vi "RIMP.vi"(2 "Run uninterrupted?":bool, 3 "Device Category IN:":string(combo)="Mini" caption="Device Category:", 4 "Batch No. IN:":string caption="Batch No.:", 5 "Sensor Serial No. IN:":string caption="Sensor Serial No.:", 6 "DB Serial No. IN:":string caption="DB Serial No.:") -> (0 "Done!":bool)   [LabVIEW 2019]
doc: "Performs IV measurements according to ATLAS ITk Quality Control Specifications."
uses:
  InstrControl/SupplyControl/SupplyControl.lvclass
  general_VIs/globals/QC_RunInformation.vi
  InstrControl/ArduinoControl/ArduinoControl.lvclass
  general_VIs/globals/QC_MeasurementSetup.vi
  <vilib>/Analysis/NI_AALBase.lvlib
  InstrControl/InstrumentSetup.vi
  InstrControl/InstrControl.lvclass
  InstrControl/Switching/Switching.lvclass
panel:
  out "Measurement Configuration Tab":enum32{"IV Setup", "IV Scan"}(tab)
  in  "Set current limit?":bool
  in  "Current Limit [µA]":dbl=1000.0 min=0.0001 format="%.3f"
  in  "Measurement Configurations":bool
  in  "Initial volts [V] IN":dbl caption="Initial volts [V]"
  in  "Final volts [V] IN":dbl=-700.0 caption="Final volts [V]"
  in  "step [V] IN":dbl=10.0 caption="step [V]" format="%.1f"
  in  "step interval [s] IN":i32=10 caption="step interval [s]"
  in  "Continue":bool
  in  "Quit":bool
  out "RH":dbl[](array[numeric]) caption="RH [%]" format="%#.2f"
  out "Temp.":dbl[](array[numeric]) caption="Temp. [°C]" format="%#.2f"
  out "Current":dbl[](array[numeric]) caption="Current [nA]"
  out "Volts":dbl[](array[numeric]) caption="Volts [V]"
  out "step interval [s]":i32=10
  out "step [V]":dbl=10.0 format="%.1f"
  out "Final volts [V]":dbl=-700.0 format="%.1f"
  out "Initial volts [V]":dbl format="%.1f"
  out "Igraph":cluster{dbl[], dbl[]}(graph)
  in  "Scales":T1(ring)
  in  "Iscale":enum16{"nanoAmps", "microAmps", "milliAmps"}(ring)
  out "positive ramp?":bool
  out "DUT Description/Hardware Tab":enum32{"IV Setup", "IV Scan"}(tab)
  in  "Structure Name IN:":string caption="Structure Name:"
  in  "Switching":string(combo)="LXIPXI Switching"
  in  "Hardware Configurations":bool
  in  "User:":string(combo)="Xavi"
  in  "IV Supply":string(combo)="Keithley 2410"
  in  "Temperature":enum16{"Read Arduino", "Enter manually"}(ring)
  in  "Manufacturer:":string(combo)="Hamamatsu"
  out "Structure Name":string caption="Structure Name:"
  in  "abort":bool
  out "Device Category:":string
  out "DB Serial No.:":string
  out "Current Volts:":dbl format="%.2f"
  in  "quit (no save)":bool
  in  "Quit & Save":bool
  out "Bias On/Off:":bool
  out "STATUS 1":string
  out "Initiated:":string
  out "Sensor No.:":string
  out "No of steps":u32
  out "Current reading No.":u32
  out "Last reading at:":string
  # "University of\nCambridge"
  # "Strip Sensor QC: Implant Resistance"
  # "Vertical Scale:"
  # "Measurement Configuration"
  # "Scan parameters:"
  # "Last 5 readings:"
  # "n-4"
  # "n-3"
  # "n-2"
  # "n-1"
  # "n"
  # "DUT Description"
  # "Hardware"
  # "DUT & Test Description:"
  # "Current status:"
  # "Rdg No:"
  # "out of"
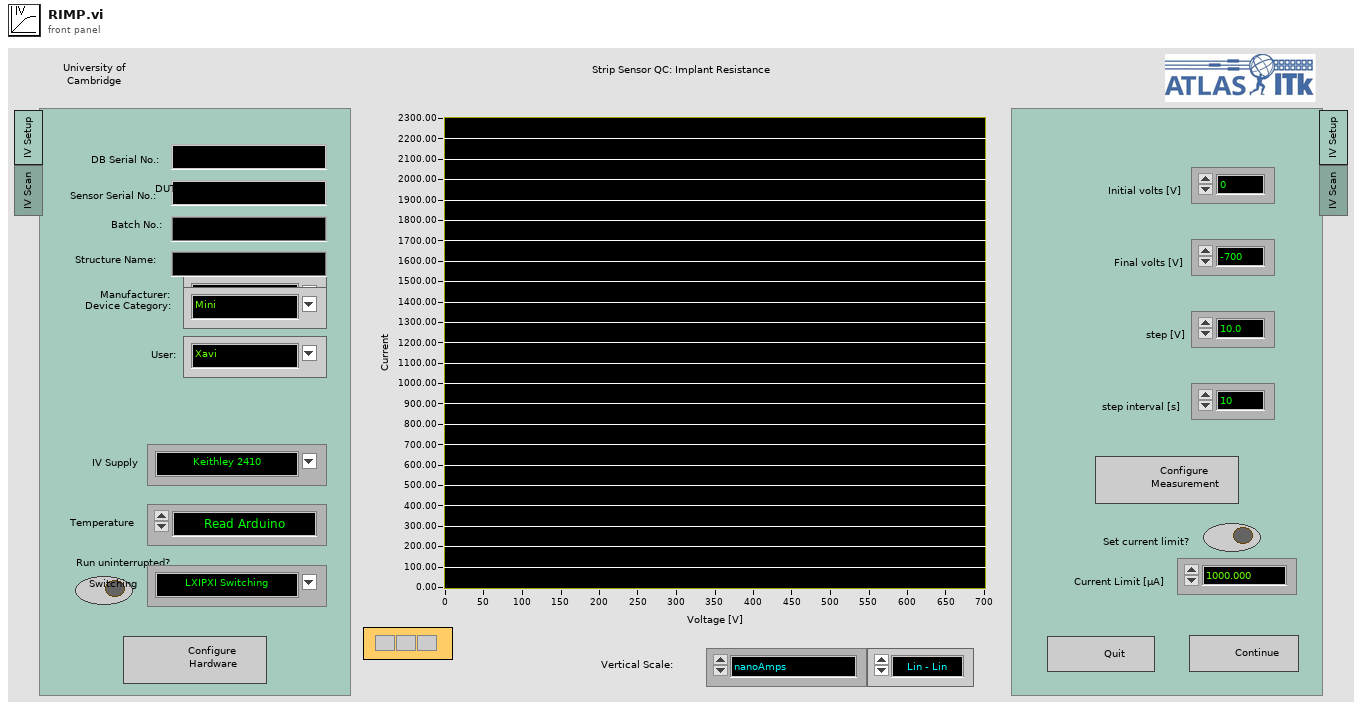
[diagram p1: front panel]
types:
  T1 = enum16{"Lin - Lin", "Log - Lin", "Lin - Log", "Log - log"}
  T2 = enum16{"Supply", "LCR", "Multimeter", "Switching"}
  T3 = enum16{"Reset", "Read Array", "Read Element", "Write Element", "Write Array", "Add Element", "Add Array"}
  T4 = enum16{"Reset", "Ground", "Striptest Bias", "Striptest SMU", "Striptest LCR", "IV", "CV", "Interstrip Cap", "Interstrip Res"}
  T5 = enum32{"IV", "CV", "Stability", "Striptest", "Cis", "Ris", "PTP"}
  T6 = cluster{"Supply":refnum<class "SupplyControl.lvclass">, "Initial Voltage [V]":dbl, "Final Voltage [V]":dbl, "Step Size [V]":dbl, "Step Interval [s]":i32, "Number Of Steps":u32, "Ramp down steps [V]":dbl, "Ramp down Interval [s]":i32, "Set Current Limit?":bool, "Current Limit [µA]":dbl, "Temperature Readout":enum16{"Read Arduino", "Enter manually"}, "Arduino":refnum<class "ArduinoControl.lvclass">, "Supply Name":string, "Switching":refnum<class "Switching.lvclass">, "Matrix used?":bool, "Matrix X Channels":cluster{"Bias Supply / SMU LO":i32, "Bias Supply / SMU HI":i32, "CV Box LO":i32, "CV Box HI":i32, "CV Box LO IN":i32, "CV Box HI IN":i32, "Volt meter LO":i32, "Volt meter HI":i32, "Mux1 C1":i32, "Mux1 C2":i32, "Mux2 C1":i32, "Mux2 C2":i32}, "Structure Name":string}
  T7 = cluster{"Sensor Serial No.:":string, "Wafer Serial No.:":string, "Batch:":string, "Manufacturer:":string, "Device Category:":string, "Database Serial No.:":string, "Date Initiated:":string, "Time Initiated:":string, "Test":string, "Instruments used:":string, "Probeplan used:":string, "End of Run comment:":string, "User:":string}
  T8 = cluster{"Institute":string, "Manufacturers":string[], "Devices":string[], "Serialnumbers Lookup DB":string, "Data directory":string, "Backup & screenshot directory":string, "List of known users":string[], "Measurement switch not used":bool, "Measurement Switch":string, "DUT Switch":string}
  T9 = cluster{"VISA address":refnum<visa-resource-name>, "T sensor":enum16{"SHT", "DS"}, "Arduino":refnum<class "ArduinoControl.lvclass">}
  T10 = cluster{"Supply":refnum<class "SupplyControl.lvclass">, "Initial Voltage [V]":dbl, "Final Voltage [V]":dbl, "Step Size [V]":dbl, "Step Interval [s]":i32, "Number Of Steps":u32, "Ramp down steps [V]":dbl, "Ramp down Interval [s]":i32, "hold steps":i32, "Set Current Limit?":bool, "Current Limit [µA]":dbl, "Temperature Readout":enum16{"Read Arduino", "Enter manually"}, "Arduino":refnum<class "ArduinoControl.lvclass">, "Supply Name":string, "V_breakdown Limit [V]":dbl, "Switching":refnum<class "Switching.lvclass">, "Matrix used?":bool, "Matrix X Channels":cluster{"Bias Supply / SMU LO":i32, "Bias Supply / SMU HI":i32, "CV Box LO":i32, "CV Box HI":i32, "CV Box LO IN":i32, "CV Box HI IN":i32, "Volt meter LO":i32, "Volt meter HI":i32, "Mux1 C1":i32, "Mux1 C2":i32, "Mux2 C1":i32, "Mux2 C2":i32}}
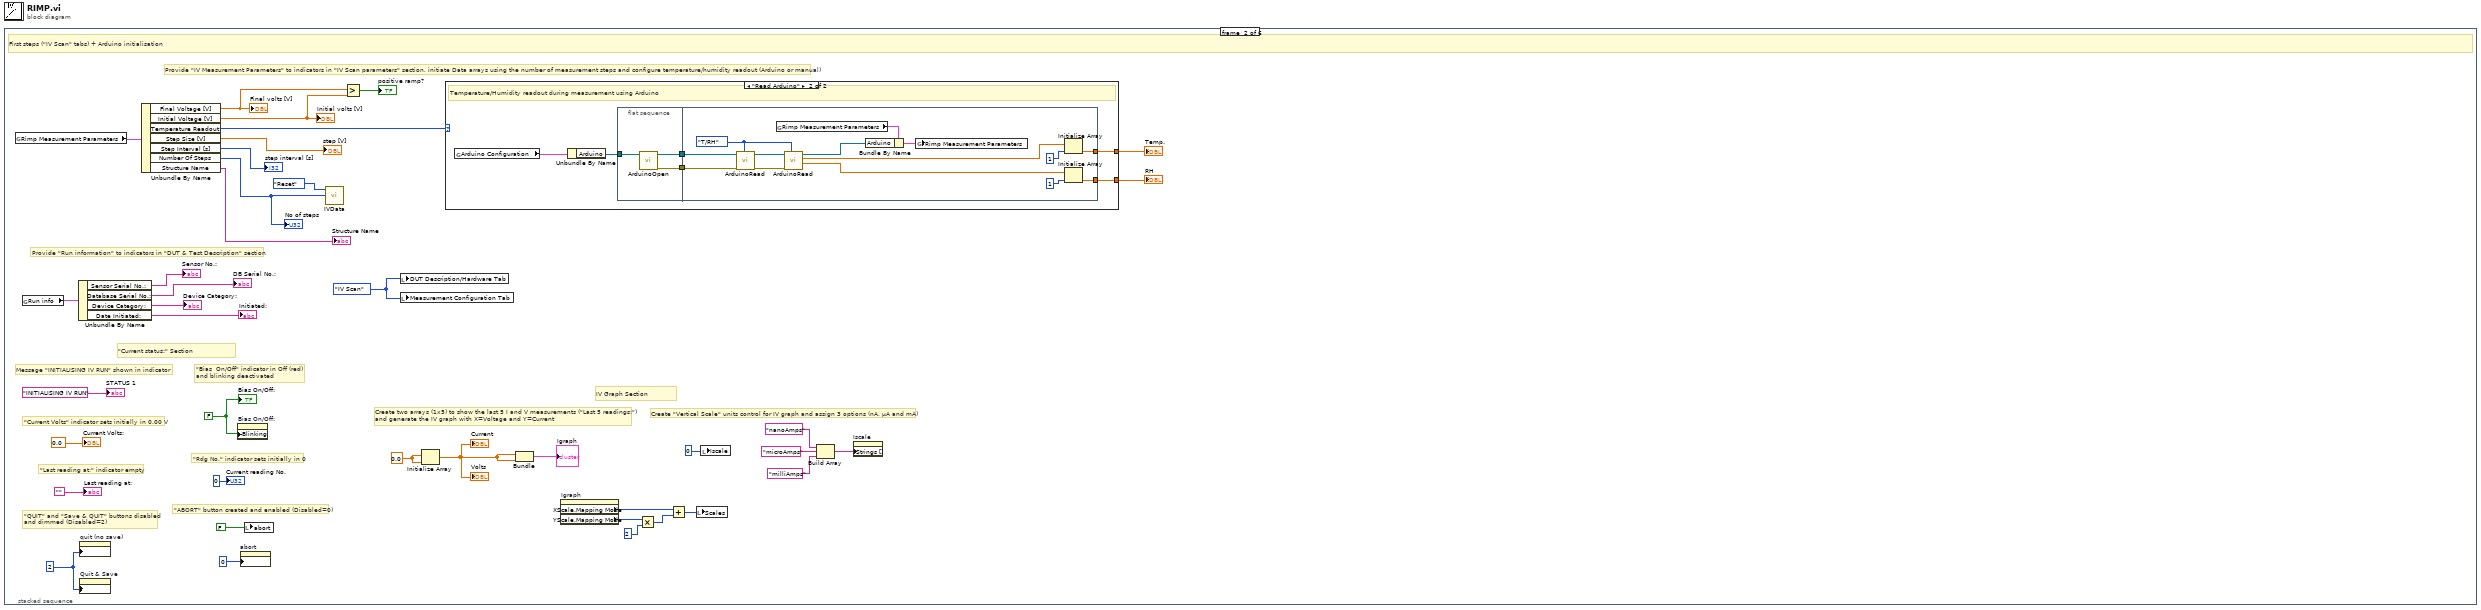
[diagram p0: block diagram]
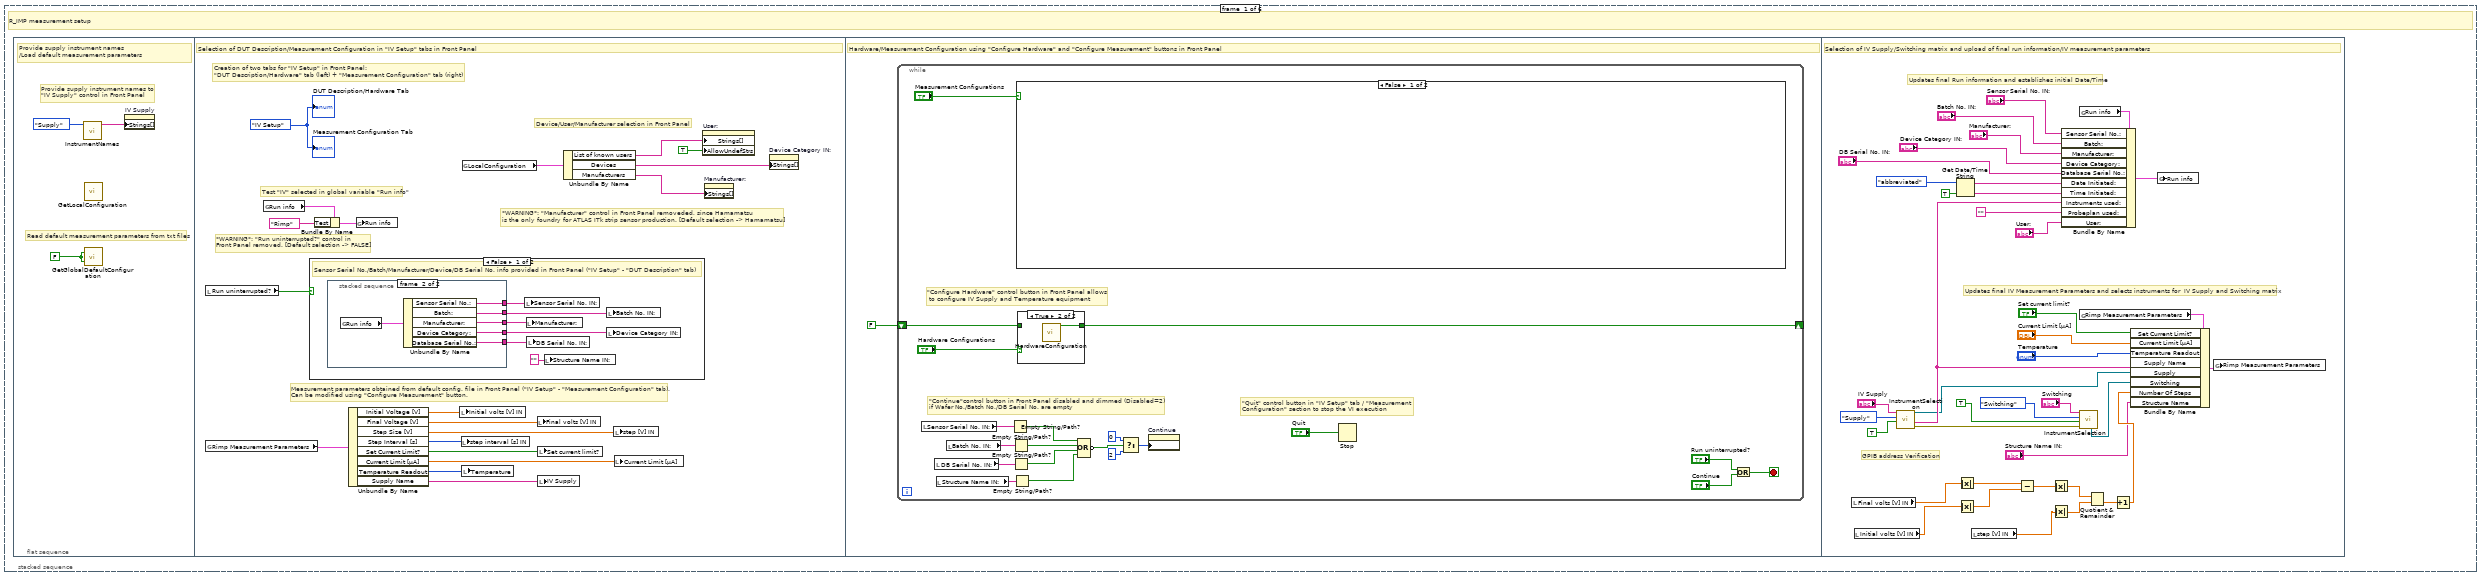
[diagram p2: hidden frame]
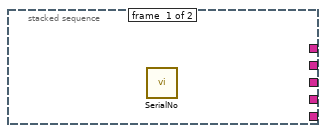
[diagram p3: hidden frame]
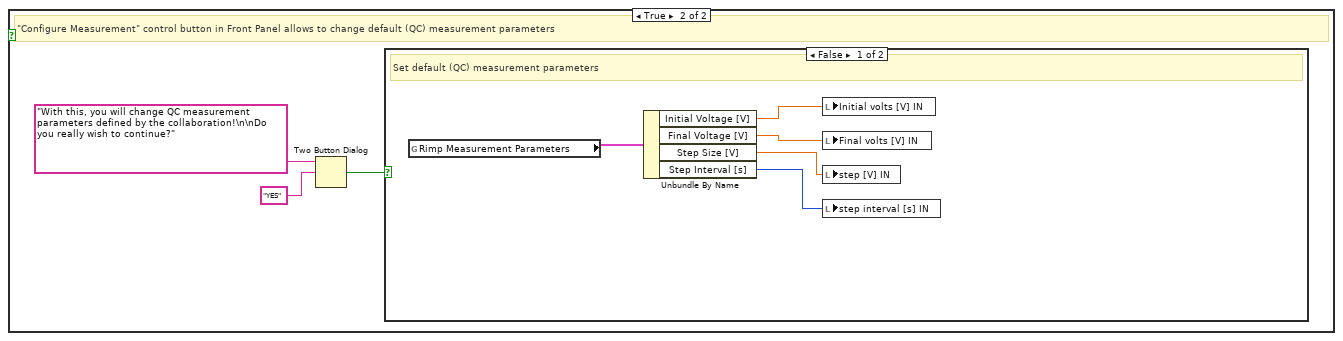
[diagram p5: hidden frame]
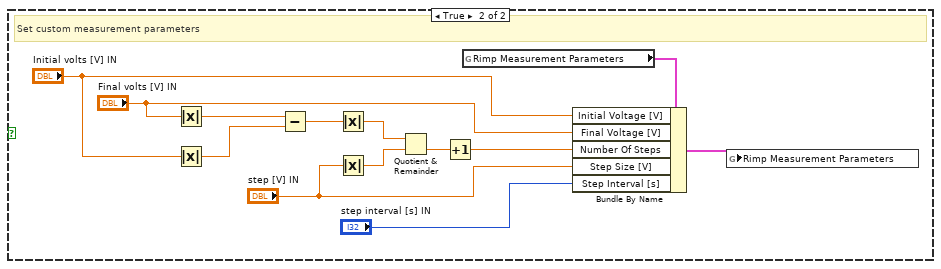
[diagram p6: hidden frame]
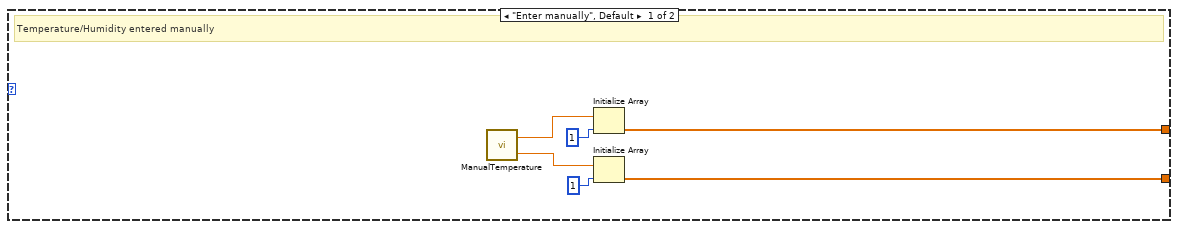
[diagram p8: hidden frame]
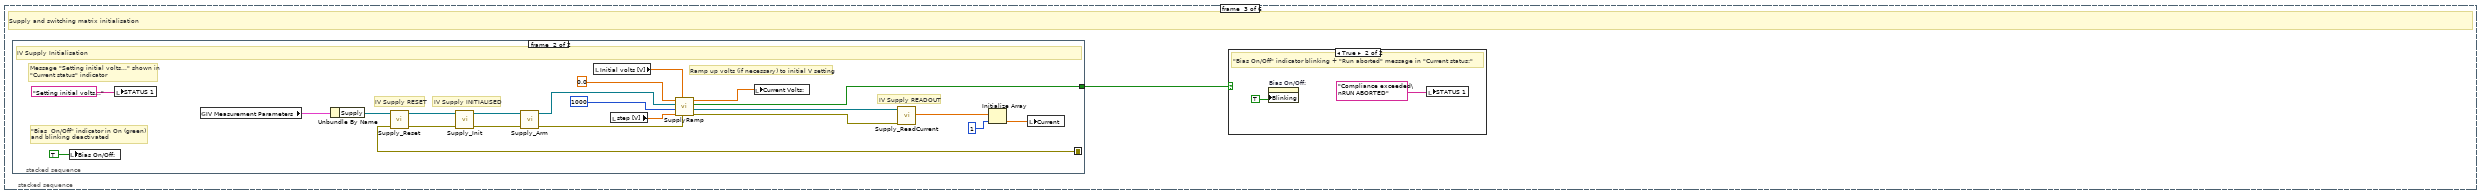
[diagram p9: hidden frame]
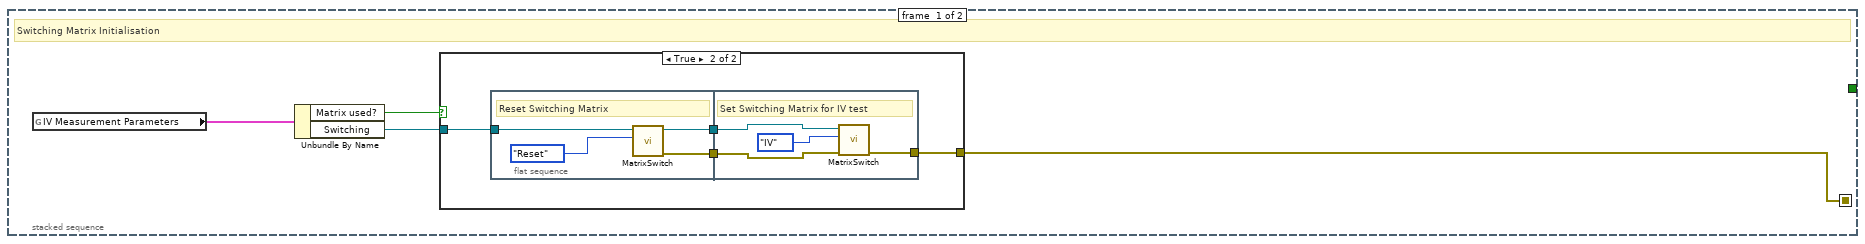
[diagram p10: hidden frame]
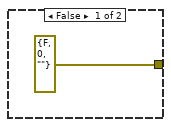
[diagram p11: hidden frame]
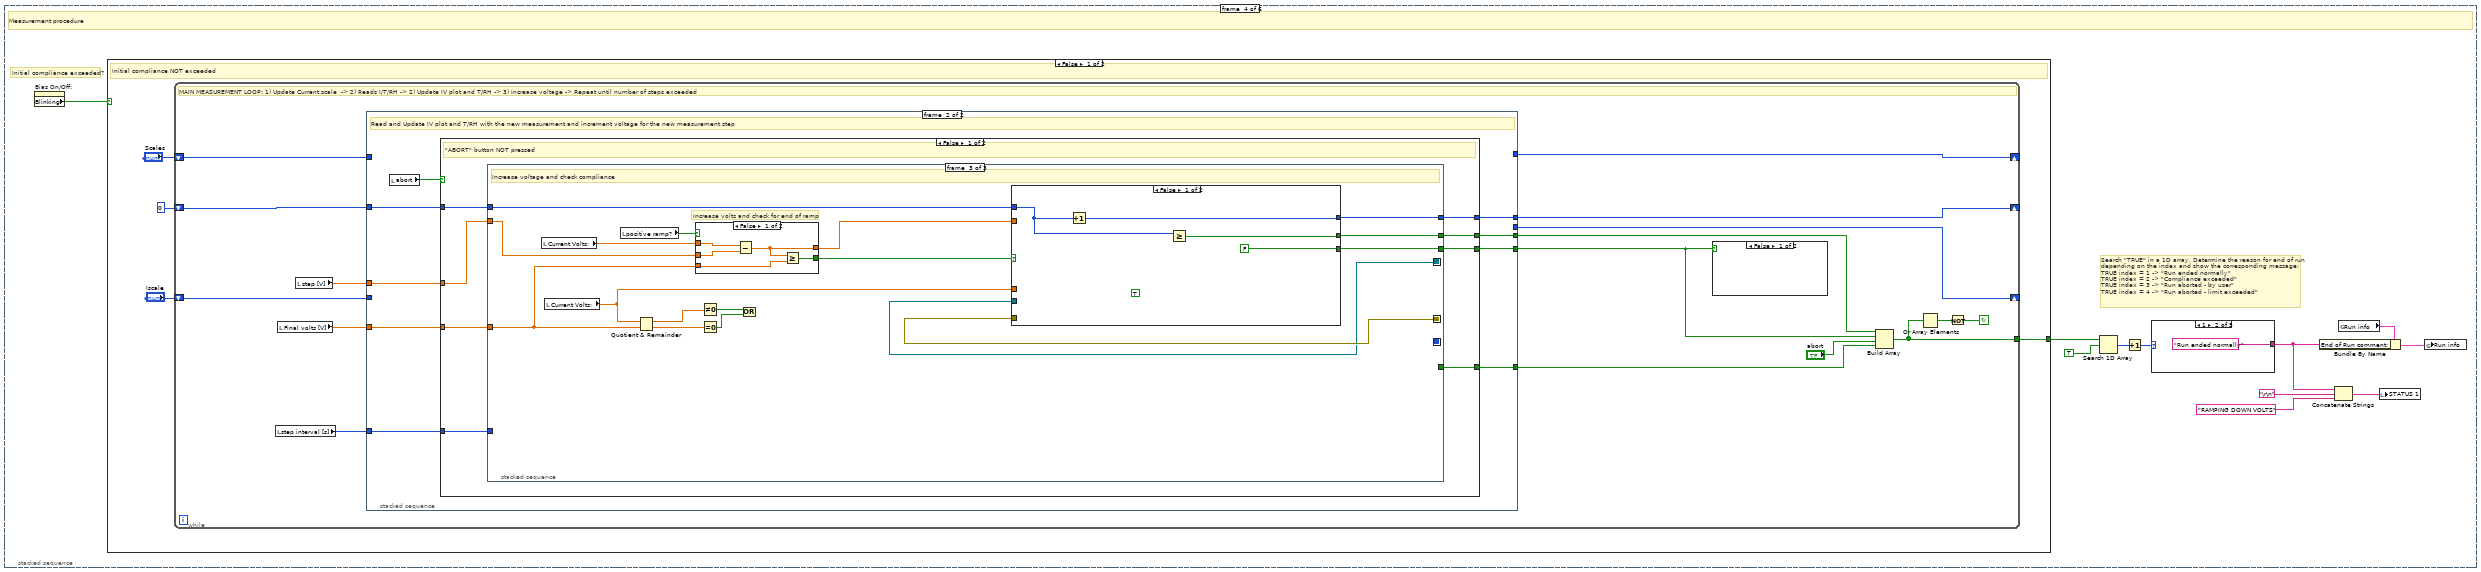
[diagram p13: hidden frame]
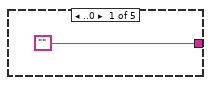
[diagram p14: hidden frame]
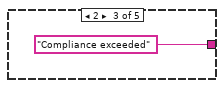
[diagram p15: hidden frame]
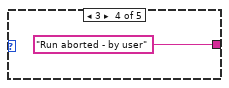
[diagram p16: hidden frame]
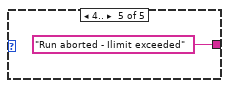
[diagram p17: hidden frame]
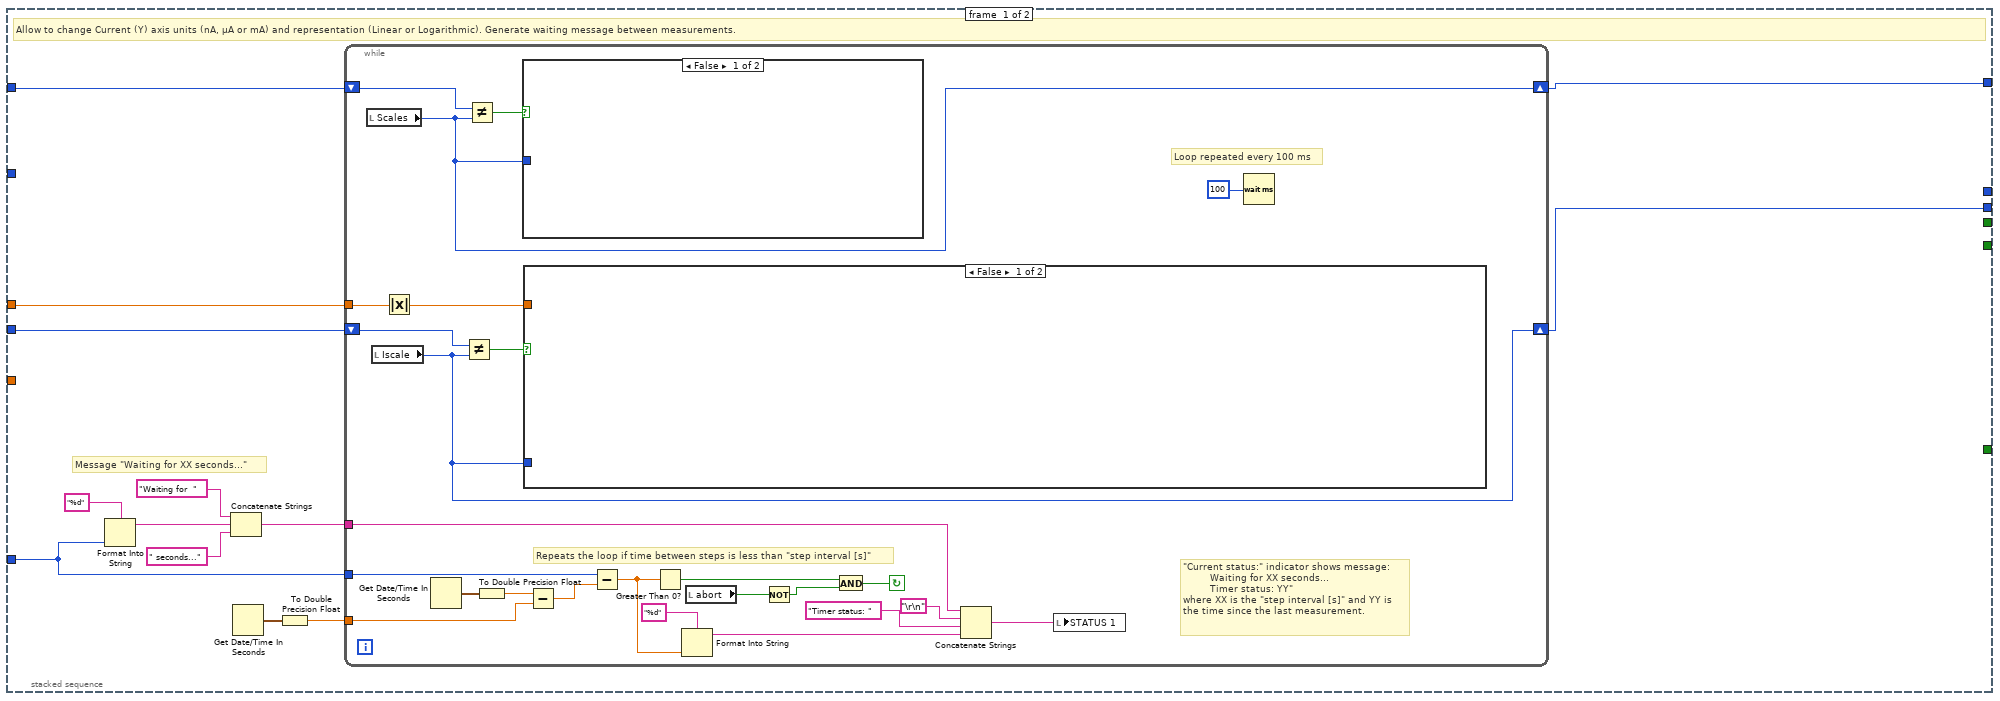
[diagram p18: hidden frame]
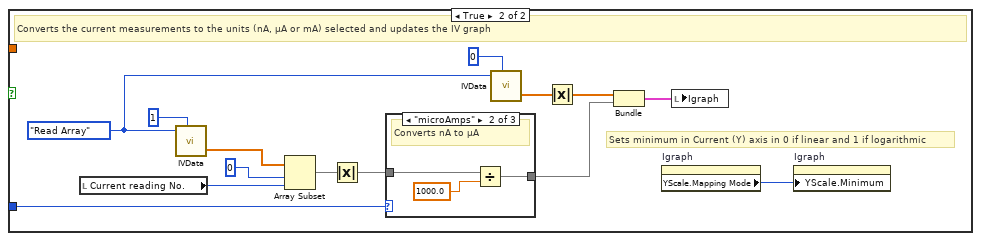
[diagram p19: hidden frame]
diagram:
  n1 = stacked-sequence {
    frame #0 {
      # "R_IMP measurement setup"
      n2 = flat-sequence {
        frame #0 {
          w3 = FALSE
          # "Read default measurement parameters from txt files"
          # "Provide supply instrument names to \n\"IV Supply\" control in Front Panel"
          # "Provide supply instrument names\n/Load default measurement parameters"
          n3 = call "InstrumentNames.vi"("Instrument type"=T2."Supply") -> ("Instrument names"=w1:string[])  [unwired: 9 in, 1 out]
          n4 = call "GetLocalConfiguration.vi"() -> ()  [unwired: 3 in, 1 out]
          n5 = call "GetGlobalDefaultConfiguration.vi"("DO NOT override instruments"=w3, "Read defaults?"=w3) -> ()  [unwired: 1 in, 1 out]
          n6 = property on="IV Supply" class="CmbBox"("Strings[]"=w1) -> ()  [unwired: 2 in, 2 out]
        }
        frame #1 {
          w11 = enum32{"IV Setup", "IV Scan"}."IV Setup" ("Tab Control")
          # "Device/User/Manufacturer selection in Front Panel"
          # "*WARNING*: \"Manufacturer\" control in Front Panel removeded, since Hamamatsu \nis the only foundry for ATLAS ITk strip sensor production. [Default selection -> Hamamatsu]"
          # "Measurement parameters obtained from default config. file in Front Panel (\"IV Setup\" - \"Measurement Configuration\" tab).\nCan be modified using \"Configure Measurement\" button."
          # "Test \"IV\" selected in global variable \"Run info\""
          # "Creation of two tabs for \"IV Setup\" in Front Panel:\n\"DUT Description/Hardware\" tab (left) + \"Measurement Configuration\" tab (right)"
          # "*WARNING*: \"Run uninterrupted?\" control in \nFront Panel removed. [Default selection -> FALSE]"
          # "Selection of DUT Description/Measurement Configuration in \"IV Setup\" tabs in Front Panel"
          n7 = local read "Run uninterrupted?"() -> (w14:bool)
          n8 = global read "QC_MeasurementSetup.vi" "Rimp Measurement Parameters"() -> (w20:T6)
          n9 = global read "QC_RunInformation.vi" "Run info"() -> (w13:T7)
          n10 = case shown="False" w14 {
            frame False {
              # "Sensor Serial No./Batch/Manufacturer/Device/DB Serial No. info provided in Front Panel (\"IV Setup\" - \"DUT Description\" tab)"
              n11 = stacked-sequence {
                tunnel: [_ w34] -> w27
                tunnel: [_ w33] -> w26
                tunnel: [_ w32] -> w25
                tunnel: [_ w31] -> w28
                tunnel: [_ w29] -> w24
                frame #0 {
                  n12 = call "SerialNo.vi"() -> ()  [unwired: 5 in, 1 out]
                }
                frame #1 {
                  n13 = global read "QC_RunInformation.vi" "Run info"() -> (w30:T7)
                  n14 = Unbundle By Name(w30) -> ("Sensor Serial No.:"=w34:string, "Batch:"=w33:string, "Manufacturer:"=w32:string, "Device Category:"=w31:string, "Database Serial No.:"=w29:string)
                }
              }
              n15 = local write "Sensor Serial No. IN:"(w27) -> ()
              n16 = local write "Manufacturer:"(w25) -> ()
              n17 = local write "DB Serial No. IN:"(w24) -> ()
              n18 = local write "Structure Name IN:"("" ("Structure Name IN:")) -> ()
              n19 = local write "Batch No. IN:"(w26) -> ()
              n20 = local write "Device Category IN:"(w28) -> ()
            }
            frame True {
            }
          }
          n21 = Bundle By Name(cluster=w13, "Test"="Rimp") -> (w12:T7)
          n22 = Unbundle By Name(w20) -> ("Initial Voltage [V]"=w9:dbl, "Final Voltage [V]"=w8:dbl, "Step Size [V]"=w7:dbl, "Step Interval [s]"=w10:i32, "Set Current Limit?"=w19:bool, "Current Limit [µA]"=w18:dbl, "Temperature Readout"=w22:enum16{"Read Arduino", "Enter manually"}, "Supply Name"=w21:string)
          n23 = global write "QC_RunInformation.vi" "Run info"(w12) -> ()
          n24 = local write "Initial volts [V] IN"(w9) -> ()
          n25 = local write "step interval [s] IN"(w10) -> ()
          n26 = local write "Temperature"(w22) -> ()
          n27 = global read "QC_RunInformation.vi" "LocalConfiguration"() -> (w17:T8)
          n28 = local write "Final volts [V] IN"(w8) -> ()
          n29 = local write "Set current limit?"(w19) -> ()
          n30 = local write "IV Supply"(w21) -> ()
          n31 = Unbundle By Name(w17) -> ("List of known users"=w16:string[], "Devices"=w6:string[], "Manufacturers"=w5:string[])
          n32 = local write "step [V] IN"(w7) -> ()
          n33 = local write "Current Limit [µA]"(w18) -> ()
          n34 = property on="User:" class="CmbBox"("Strings[]"=w16, "AllowUndefStrs"=TRUE) -> ()  [unwired: 2 in, 2 out]
          n35 = property on="Manufacturer:" class="CmbBox"("Strings[]"=w5) -> ()  [unwired: 2 in, 2 out]
          n36 = property on="Device Category IN:" class="CmbBox"("Strings[]"=w6) -> ()  [unwired: 2 in, 2 out]
          "DUT Description/Hardware Tab" <- w11
          "Measurement Configuration Tab" <- w11
        }
        frame #2 {
          # "Hardware/Measurement Configuration using \"Configure Hardware\" and \"Configure Measurement\" buttons in Front Panel"
          n37 = while {
            shift-right: [w45] -> _
            shift-left: FALSE -> [w44]
            stop <- w41 stop-if-true
            # "\"Continue\"control button in Front Panel disabled and dimmed (Disabled=2) \nif Wafer No./Batch No./DB Serial No. are empty"
            # "\"Configure Hardware\" control button in Front Panel allows\n to configure IV Supply and Temperature equipment"
            # "\"Quit\" control button in \"IV Setup\" tab / \"Measurement \nConfiguration\" section to stop the VI execution"
            n38 = local read "Sensor Serial No. IN:"() -> (w54:string)
            n39 = local read "DB Serial No. IN:"() -> (w39:string)
            n40 = local read "Structure Name IN:"() -> (w37:string)
            n41 = local read "Batch No. IN:"() -> (w47:string)
            n42 = Empty String/Path?(string/path=w54) -> (empty?=w53:bool)
            n43 = Empty String/Path?(string/path=w47) -> (empty?=w46:bool)
            n44 = Empty String/Path?(string/path=w39) -> (empty?=w38:bool)
            n45 = Empty String/Path?(string/path=w37) -> (empty?=w36:bool)
            n46 = case shown="False" "Measurement Configurations" {
              frame False {
              }
              frame True {
                # "\"Configure Measurement\" control button in Front Panel allows to change default (QC) measurement parameters"
                n47 = Two Button Dialog(message="With this, you will change QC measurement parameters defined by the collaboration!\n\nDo you really wish to continue?", 2:"YES") -> (T button?=w56:bool)  [unwired: 1 in]
                n48 = case shown="False" w56 {
                  frame False {
                    # "Set default (QC) measurement parameters"
                    n49 = global read "QC_MeasurementSetup.vi" "Rimp Measurement Parameters"() -> (w63:T6)
                    n50 = Unbundle By Name(w63) -> ("Initial Voltage [V]"=w61:dbl, "Final Voltage [V]"=w62:dbl, "Step Size [V]"=w60:dbl, "Step Interval [s]"=w59:i32)
                    n51 = local write "Initial volts [V] IN"(w61) -> ()
                    n52 = local write "Final volts [V] IN"(w62) -> ()
                    n53 = local write "step [V] IN"(w60) -> ()
                    n54 = local write "step interval [s] IN"(w59) -> ()
                  }
                  frame True {
                    # "Set custom measurement parameters"
                    n55 = Absolute Value(x="Final volts [V] IN") -> (abs(x)=w74:dbl)
                    n56 = Absolute Value(x="Initial volts [V] IN") -> (abs(x)=w73:dbl)
                    n57 = Subtract(x=w74, y=w73) -> (x-y=w68:dbl)
                    n58 = Absolute Value(x=w68) -> (abs(x)=w70:dbl)
                    n59 = Absolute Value(x="step [V] IN") -> (abs(x)=w69:dbl)
                    n60 = Quotient & Remainder(x=w70, y=w69) -> (floor(x/y)=w67:dbl)  [unwired: 1 out]
                    n61 = Increment(x=w67) -> (x+1=w66:dbl)
                    n62 = global read "QC_MeasurementSetup.vi" "Rimp Measurement Parameters"() -> (w76:T6)
                    n63 = Bundle By Name(cluster=w76, "Initial Voltage [V]"="Initial volts [V] IN", "Final Voltage [V]"="Final volts [V] IN", "Number Of Steps"=w66, "Step Size [V]"="step [V] IN", "Step Interval [s]"="step interval [s] IN") -> (w75:T6)
                    n64 = global write "QC_MeasurementSetup.vi" "Rimp Measurement Parameters"(w75) -> ()
                  }
                }
              }
            }
            n65 = case shown="True" "Hardware Configurations" {
              tunnel: [w77 w78] -> w45
              tunnel: w44 -> [w77 _]
              frame False {
              }
              frame True {
                n66 = call "HardwareConfiguration.vi"() -> ("configured?"=w78:bool)  [unwired: 11 in]
              }
            }
            n67 = Compound Arithmetic op=OR(w53, w46, w38, w36) -> (invert w52:bool)
            n68 = Select(t=0, s=w52, f=2) -> (s? t:f=w49:i32)
            n69 = property on="Continue" class="Bool"("DisabledEnum"=w49) -> ()  [unwired: 2 in, 2 out]
            n70 = Stop(stop? (T)="Quit") -> ()
            n71 = Or(x="Run uninterrupted?", y="Continue") -> (x .or. y?=w41:bool)
          }
        }
        frame #3 {
          # "GPIB address Verification"
          # "Updates final IV Measurement Parameters and selects instruments for  IV Supply and Switching matrix"
          # "Updates final Run information and establishes initial Date/Time"
          # "Selection of IV Supply/Switching matrix and upload of final run information/IV measurement parameters"
          n72 = local read "Final volts [V] IN"() -> (w81:dbl)
          n73 = local read "Initial volts [V] IN"() -> (w82:dbl)
          n74 = call "InstrumentSelection.vi"("Verify GPIB address"=TRUE, "Instrument type"=T2."Supply", "Instrument name IN"="IV Supply") -> ("error out"=w100:errorcluster, "Instrument name OUT"=w103:string, "Supply"=w102:refnum<class "SupplyControl.lvclass">)  [unwired: 3 in, 3 out]
          n75 = Get Date/Time String(date format (0)=enum16{"short", "long", "abbreviated"}."abbreviated", want seconds? (F)=TRUE) -> (date string=w93:string, time string=w92:string)  [unwired: 1 in]
          n76 = Absolute Value(x=w81) -> (abs(x)=w89:dbl)
          n77 = Absolute Value(x=w82) -> (abs(x)=w88:dbl)
          n78 = local read "step [V] IN"() -> (w83:dbl)
          n79 = Subtract(x=w89, y=w88) -> (x-y=w85:dbl)
          n80 = Absolute Value(x=w85) -> (abs(x)=w87:dbl)
          n81 = Absolute Value(x=w83) -> (abs(x)=w86:dbl)
          n82 = global read "QC_RunInformation.vi" "Run info"() -> (w111:T7)
          n83 = Bundle By Name(cluster=w111, "Sensor Serial No.:"="Sensor Serial No. IN:", "Batch:"="Batch No. IN:", "Manufacturer:"="Manufacturer:", "Device Category:"="Device Category IN:", "Database Serial No.:"="DB Serial No. IN:", "Date Initiated:"=w93, "Time Initiated:"=w92, "Instruments used:"=w103, "Probeplan used:"="", "User:"="User:") -> (w110:T7)
          n84 = global read "QC_MeasurementSetup.vi" "Rimp Measurement Parameters"() -> (w116:T6)
          n85 = call "InstrumentSelection.vi"("error in (no error)"=w100, "Verify GPIB address"=TRUE, "Instrument type"=T2."Switching", "Instrument name IN"="Switching") -> ("Switching"=w99:refnum<class "Switching.lvclass">)  [unwired: 2 in, 5 out]
          n86 = Quotient & Remainder(x=w87, y=w86) -> (floor(x/y)=w84:dbl)  [unwired: 1 out]
          n87 = Increment(x=w84) -> (x+1=w80:dbl)
          n88 = Bundle By Name(cluster=w116, "Set Current Limit?"="Set current limit?", "Current Limit [µA]"="Current Limit [µA]", "Temperature Readout"="Temperature", "Supply Name"=w103, "Supply"=w102, "Switching"=w99, "Number Of Steps"=w80, "Structure Name"="Structure Name IN:") -> (w117:T6)
          n89 = global write "QC_RunInformation.vi" "Run info"(w110) -> ()
          n90 = global write "QC_MeasurementSetup.vi" "Rimp Measurement Parameters"(w117) -> ()
        }
      }
    }
    frame #1 {
      w125 = enum32{"IV Setup", "IV Scan"}."IV Scan" ("Tab Control")
      w140 = 2
      w146 = 0.0
      w139 = FALSE ("Visible")
      # "IV Graph Section"
      # "\"Current status:\" Section"
      # "Create two arrays (1x5) to show the last 5 I and V measurements (\"Last 5 readings:\") \nand generate the IV graph with X=Voltage and Y=Current"
      # "\"Bias  On/Off\" indicator in Off (red)\nand blinking deactivated"
      # "\"Rdg No.\" indicator sets initially in 0"
      # "\"ABORT\" button created and enabled (Disabled=0)"
      # "\"Current Volts\" indicator sets initially in 0.00 V"
      # "\"Last reading at:\" indicator empty"
      # "\"QUIT\" and \"Save & QUIT\" buttons disabled\nand dimmed (Disabled=2)"
      # "Message \"INITIALISING IV RUN\" shown in indicator"
      # "Create \"Vertical Scale\" units control for IV graph and assign 3 options (nA, µA and mA)"
      # "Provide \"Run information\" to indicators in \"DUT & Test Description\" section"
      # "Provide \"IV Measurement Parameters\" to indicators in \"IV Scan parameters\" section, initiate Data arrays using the number of measurement steps and configure temperature/humidity readout (Arduino or manual)"
      # "First steps (\"IV Scan\" tabs) + Arduino initialisation"
      n91 = global read "QC_MeasurementSetup.vi" "Rimp Measurement Parameters"() -> (w130:T6)
      n92 = global read "QC_RunInformation.vi" "Run info"() -> (w155:T7)
      n93 = Unbundle By Name(w155) -> ("Sensor Serial No.:"=→"Sensor No.:":string, "Database Serial No.:"=→"DB Serial No.:":string, "Device Category:"=→"Device Category:":string, "Date Initiated:"=→"Initiated:":string)
      n94 = property on="quit (no save)" class="Bool"("DisabledEnum"=w140) -> ()  [unwired: 2 in, 2 out]
      n95 = property on="Quit & Save" class="Bool"("DisabledEnum"=w140) -> ()  [unwired: 2 in, 2 out]
      n96 = Unbundle By Name(w130) -> ("Final Voltage [V]"=w121:dbl, "Initial Voltage [V]"=w122:dbl, "Temperature Readout"=w123:enum16{"Read Arduino", "Enter manually"}, "Step Size [V]"=→"step [V]":dbl, "Step Interval [s]"=→"step interval [s]":i32, "Number Of Steps"=w119:u32, "Structure Name"=→"Structure Name":string)
      "No of steps" <- w119
      "Initial volts [V]" <- w122
      "Final volts [V]" <- w121
      n97 = property on="Bias On/Off:" class="Bool (strict)"("Blinking"=w139) -> ()  [unwired: 2 in, 2 out]
      n98 = property on="abort" class="Bool (strict)"("DisabledEnum"=0) -> ()  [unwired: 2 in, 2 out]
      n99 = local write "abort"(FALSE) -> ()
      n100 = call "IVData.vi"("Action"=T3."Reset", "Array Size / Index"=w119) -> ()  [unwired: 3 in, 2 out]
      n101 = Greater?(x=w121, y=w122) -> (0:→"positive ramp?":bool)
      n102 = local write "DUT Description/Hardware Tab"(w125) -> ()
      n103 = local write "Measurement Configuration Tab"(w125) -> ()
      n104 = Initialize Array(w146, w146) -> (w126:dbl[])
      "Volts" <- w126
      "Current" <- w126
      n105 = case shown="\"Read Arduino\"" w123 {
        tunnel: [w161 w168] -> w143
        tunnel: [w158 w167] -> w131
        frame "Enter manually", Default {
          # "Temperature/Humidity entered manually"
          n106 = call "ManualTemperature.vi"() -> ("Humidity [%] out"=w157:dbl, "Temperature [°C] out"=w162:dbl)
          n107 = Initialize Array(w162, 1) -> (w161:dbl[])
          n108 = Initialize Array(w157, 1) -> (w158:dbl[])
        }
        frame "Read Arduino" {
          # "Temperature/Humidity readout during measurement using Arduino"
          n109 = global read "InstrumentSetup.vi" "Arduino Configuration"() -> (w164:T9)
          n110 = Unbundle By Name(w164) -> ("Arduino"=w163:refnum<class "ArduinoControl.lvclass">)
          n111 = flat-sequence {
            tunnel: [w169] -> w166
            tunnel: [w171] -> w165
            tunnel: w163 -> [w170]
            tunnel: [w185] -> w168
            tunnel: [w182] -> w167
            tunnel: w166 -> [w176]
            tunnel: w165 -> [w175]
            frame #0 {
              n112 = call "ArduinoOpen.vi"("ArduinoControl in"=w170) -> ("error out"=w171:errorcluster, "ArduinoControl out"=w169:refnum<class "ArduinoControl.lvclass">)  [unwired: 9 in]
            }
            frame #1 {
              w172 = enum16{"T/RH", "Interlock", "Edgesense"}."T/RH" ("Arduino function")
              n113 = call "ArduinoRead.vi"("Arduino function"=w172, "error in (no error)"=w175, "ArduinoControl in"=w176) -> ("error out"=w174:errorcluster, "ArduinoControl out"=w173:refnum<class "ArduinoControl.lvclass">)  [unwired: 3 in, 4 out]
              n114 = global read "QC_MeasurementSetup.vi" "Rimp Measurement Parameters"() -> (w178:T6)
              n115 = call "ArduinoRead.vi"("Arduino function"=w172, "error in (no error)"=w174, "ArduinoControl in"=w173) -> ("rel. Humidity [%]"=w180:dbl, "Temperature [°C]"=w181:dbl, "ArduinoControl out"=w179:refnum<class "ArduinoControl.lvclass">)  [unwired: 3 in, 3 out]
              n116 = Bundle By Name(cluster=w178, "Arduino"=w179) -> (w177:T6)
              n117 = global write "QC_MeasurementSetup.vi" "Rimp Measurement Parameters"(w177) -> ()
              n118 = Initialize Array(w181, 1) -> (w185:dbl[])
              n119 = Initialize Array(w180, 1) -> (w182:dbl[])
            }
          }
        }
      }
      "Temp." <- w143
      "RH" <- w131
      n120 = Bundle(w126, w126) -> (→"Igraph":cluster{dbl[], dbl[]})  [unwired: 1 in]
      n121 = property on="Igraph" class="XYGraph (strict)"() -> ("XScale.Mapping Mode"=w134:u8, "YScale.Mapping Mode"=w133:u8)  [unwired: 2 in, 2 out]
      n122 = Multiply(x=w133, y=2) -> (x*y=w136:i32)
      n123 = Add(x=w134, y=w136) -> (x+y=w132:i32)
      n124 = local write "Scales"(w132) -> ()
      n125 = local write "Iscale"(u16 0 ("Scale")) -> ()
      n126 = Build Array("nanoAmps", "microAmps", "milliAmps") -> (w152:string[])
      n127 = property on="Iscale" class="Enum (strict)"("Strings []"=w152) -> ()  [unwired: 2 in, 2 out]
      "STATUS 1" <- "INITIALISING IV RUN"
      "Bias On/Off:" <- w139
      "Last reading at:" <- ""
      "Current reading No." <- u32 0 ("Current reading No.")
      "Current Volts:" <- 0.0 ("Current Volts:")
    }
    frame #2 {
      # "Supply and switching matrix initialisation"
      n128 = stacked-sequence {
        seq-local: [w188 _] -> [_ w204]
        tunnel: [_ w205] -> w186
        frame #0 {
          # "Switching Matrix Initialisation"
          n129 = global read "QC_MeasurementSetup.vi" "IV Measurement Parameters"() -> (w187:T10)
          n130 = Unbundle By Name(w187) -> ("Matrix used?"=w190:bool, "Switching"=w189:refnum<class "Switching.lvclass">)
          n131 = case shown="True" w190 {
            tunnel: w189 -> [_ w192]
            tunnel: [errorcluster {"status"=FALSE, "code"=0, "source"=""} ("error constant") w193] -> w188
            frame False {
            }
            frame True {
              n132 = flat-sequence {
                tunnel: [w199] -> w195
                tunnel: [w198] -> w194
                tunnel: w192 -> [w197]
                tunnel: w195 -> [w203]
                tunnel: w194 -> [w202]
                tunnel: [w201] -> w193
                frame #0 {
                  # "Reset Switching Matrix"
                  n133 = call-dynamic "MatrixSwitch.vi"("Action"=T4."Reset", "Switching in"=w197) -> ("error out"=w199:errorcluster, "Switching out"=w198:refnum<class "Switching.lvclass">)  [unwired: 7 in, 1 out]
                }
                frame #1 {
                  # "Set Switching Matrix for IV test"
                  n134 = call-dynamic "MatrixSwitch.vi"("error in (no error)"=w203, "Action"=T4."IV", "Switching in"=w202) -> ("error out"=w201:errorcluster)  [unwired: 6 in, 2 out]
                }
              }
            }
          }
        }
        frame #1 {
          # "IV Supply READOUT"
          # "IV Supply INITIALISED"
          # "IV Supply RESET"
          # "Message \"Setting initial volts...\" shown in \n\"Current status\" indicator"
          # "\"Bias  On/Off\" indicator in On (green)\nand blinking deactivated"
          # "Ramp up volts (if necessary) to initial V setting"
          # "IV Supply Initialisation"
          n135 = local write "Bias On/Off:"(TRUE ("Compliance?")) -> ()
          n136 = local write "STATUS 1"("Setting initial volts..." ("STATUS 1")) -> ()
          n137 = global read "QC_MeasurementSetup.vi" "IV Measurement Parameters"() -> (w221:T10)
          n138 = Unbundle By Name(w221) -> ("Supply"=w218:refnum<class "SupplyControl.lvclass">)
          n139 = call-dynamic "Supply_Reset.vi"("error in (no error)"=w204, "SupplyControl in"=w218) -> ("error out"=w223:errorcluster, "SupplyControl out"=w225:refnum<class "SupplyControl.lvclass">)  [unwired: 8 in]
          n140 = call-dynamic "Supply_Init.vi"("error in (no error)"=w223, "SupplyControl in"=w225) -> ("error out"=w222:errorcluster, "SupplyControl out"=w224:refnum<class "SupplyControl.lvclass">)  [unwired: 8 in]
          n141 = call-dynamic "Supply_Arm.vi"("error in (no error)"=w222, "SupplyControl in"=w224) -> ("error out"=w211:errorcluster, "SupplyControl out"=w212:refnum<class "SupplyControl.lvclass">)  [unwired: 8 in]
          n142 = local read "Initial volts [V]"() -> (w213:dbl)
          n143 = local read "step [V]"() -> (w214:dbl)
          n144 = call "SupplyRamp.vi"("error in"=w211, "Requested Voltage"=w213, "Step Size"=w214, "Step Delay"=1000, "Supply IN"=w212, "Starting Voltage"=0.0) -> ("error out"=w206:errorcluster, "Supply OUT"=w207:refnum<class "SupplyControl.lvclass">, "Compliance exceeded"=w205:bool, "Current Voltage"=w217:dbl)  [unwired: 2 in]
          n145 = local write "Current Volts:"(w217) -> ()
          n146 = call-dynamic "Supply_ReadCurrent.vi"("error in (no error)"=w206, "SupplyControl in"=w207) -> ("Current in nA"=w209:dbl)  [unwired: 7 in, 2 out]
          n147 = Initialize Array(w209, 1) -> (w208:dbl[])
          n148 = local write "Current"(w208) -> ()
        }
      }
      n149 = case shown="True" w186 {
        frame False {
        }
        frame True {
          # "\"Bias On/Off\" indicator blinking + \"Run aborted\" message in \"Current status:\""
          n150 = property on="Bias On/Off:" class="Bool (strict)"("Blinking"=TRUE) -> ()  [unwired: 2 in, 2 out]
          n151 = local write "STATUS 1"("Compliance exceeded\nRUN ABORTED") -> ()
        }
      }
    }
    frame #3 {
      # "Search \"TRUE\" in a 1D array. Determine the reason for end of run \ndepending on the index and show the corresponding message:\nTRUE index = 1 -> \"Run ended normally\"\nTRUE index = 2 -> \"Compliance exceeded\"\nTRUE index = 3 -> \"Run aborted - by user\"\nTRUE index = 4 -> \"Run aborted - limit exceeded\""
      # "Initial compliance exceeded?"
      # "Measurement procedure"
      n152 = property on="Bias On/Off:" class="Bool (strict)"() -> ("Blinking"=w238:bool)  [unwired: 2 in, 2 out]
      n153 = case shown="False" w238 {
        tunnel: [w247 w504] -> w237
        frame False {
          # "Initial compliance NOT exceeded"
          n154 = while {
            shift-left: "Iscale" -> [w259]
            shift-right: [w258] -> _
            shift-left: "Scales" -> [w260]
            shift-right: [w261] -> _
            tunnel: [w257] -> w247
            shift-right: [w249] -> _
            shift-left: 0 -> [w250]
            stop <- w262 continue-if-true
            # "MAIN MEASUREMENT LOOP: 1) Update Current scale  -> 2) Reads I/T/RH -> 2) Update IV plot and T/RH -> 3) Increase voltage -> Repeat until number of steps exceeded"
            n155 = local read "step interval [s]"() -> (w254:i32)
            n156 = local read "Final volts [V]"() -> (w255:dbl)
            n157 = local read "step [V]"() -> (w256:dbl)
            n158 = stacked-sequence {
              tunnel: [w276 _] -> w261
              tunnel: w256 -> [w273 w340]
              tunnel: [_ w339] -> w252
              tunnel: w255 -> [_ w338]
              tunnel: w254 -> [w264 w337]
              tunnel: [_ w336] -> w253
              tunnel: w260 -> [w275 _]
              tunnel: w259 -> [w274 _]
              tunnel: [w272 _] -> w258
              tunnel: [_ w334] -> w248
              tunnel: w250 -> [_ w333]
              tunnel: [_ w332] -> w249
              frame #0 {
                # "Message \"Waiting for XX seconds...\""
                # "Allow to change Current (Y) axis units (nA, µA or mA) and representation (Linear or Logarithmic). Generate waiting message between measurements."
                n159 = Format Into String(format string="%d", w264) -> (resulting string=w269:string)  [unwired: 2 in, 1 out]
                n160 = Concatenate Strings("Waiting for  ", w269, " seconds...") -> (w265:string)
                n161 = Get Date/Time In Seconds() -> (seconds since 1Jan1904=w266:timestamp)
                n162 = To Double Precision Float(number=w266) -> (double precision float=w267:dbl)
                n163 = while {
                  tunnel: w273 -> [w285]
                  shift-left: w274 -> [w289]
                  shift-right: [w282] -> w272
                  shift-left: w275 -> [w290]
                  shift-right: [w291] -> w276
                  tunnel: w265 -> [w283]
                  tunnel: w264 -> [w295]
                  tunnel: w267 -> [w296]
                  stop <- w297 continue-if-true
                  # "\"Current status:\" indicator shows message:\n         Waiting for XX seconds...\n         Timer status: YY\"\nwhere XX is the \"step interval [s]\" and YY is\nthe time since the last measurement."
                  # "Repeats the loop if time between steps is less than \"step interval [s]\""
                  # "Loop repeated every 100 ms"
                  n164 = local read "Scales"() -> (w291:T1)
                  n165 = local read "Iscale"() -> (w282:enum16{"nanoAmps", "microAmps", "milliAmps"})
                  n166 = Absolute Value(x=w285) -> (abs(x)=w284:dbl)
                  n167 = Get Date/Time In Seconds() -> (seconds since 1Jan1904=w281:timestamp)
                  n168 = Not Equal?(x=w289, y=w282) -> (x != y?=w280:bool)
                  n169 = Not Equal?(x=w290, y=w291) -> (x != y?=w292:bool)
                  n170 = To Double Precision Float(number=w281) -> (double precision float=w301:dbl)
                  n171 = case shown="False" w292 {
                    tunnel: w291 -> [_ w325]
                    frame False {
                    }
                    frame True {
                      # "Linear (0) or Logarithmical (1) representation of X and Y axis in IV graph"
                      n172 = case shown="\"Log - Lin\"" w325 {
                        tunnel: [w326 1 0 w331] -> w324
                        tunnel: [w326 0 1 w331] -> w323
                        frame .."Lin - Lin" {
                          w326 = 0
                        }
                        frame "Log - Lin" {
                        }
                        frame "Lin - Log" {
                        }
                        frame "Log - log".. {
                          w331 = 1
                        }
                      }
                      n173 = property on="Igraph" class="XYGraph (strict)"("X Scale.Mapping Mode"=w324) -> ()  [unwired: 2 in, 2 out]
                      n174 = property on="Igraph" class="XYGraph (strict)"("Y Scale.Mapping Mode"=w323, "YScale.Minimum"=w323) -> ()  [unwired: 2 in, 2 out]
                    }
                  }
                  n175 = case shown="False" w280 {
                    tunnel: w284 -> [_ _]
                    tunnel: w282 -> [_ w310]
                    frame False {
                    }
                    frame True {
                      w304 = T3."Read Array" ("Action")
                      # "Sets minimum in Current (Y) axis in 0 if linear and 1 if logarithmic"
                      # "Converts the current measurements to the units (nA, µA or mA) selected and updates the IV graph"
                      n176 = local read "Current reading No."() -> (w312:u32)
                      n177 = call "IVData.vi"("Action"=w304, "Array No."=u32 1 ("Action")) -> ("Array OUT"=w313:dbl[])  [unwired: 3 in, 1 out]
                      n178 = Array Subset(array=w313, index=0, length=w312) -> (w309:dbl[])
                      n179 = Absolute Value(x=w309) -> (abs(x)=w308:dbl[])
                      n180 = case shown="\"microAmps\"" w310 {
                        tunnel: [w316 w317 w321] -> w315
                        tunnel: w308 -> [w316 w319 w322]
                        frame .."nanoAmps" {
                        }
                        frame "microAmps" {
                          # "Converts nA to µA"
                          n181 = Divide(x=w319, y=1000.0) -> (x/y=w317:dbl[])
                        }
                        frame "milliAmps".. {
                          # "Converts nA to mA"
                          n182 = Divide(x=w322, y=1000000.0) -> (x/y=w321:dbl[])
                        }
                      }
                      n183 = call "IVData.vi"("Action"=w304, "Array No."=u32 0 ("Action")) -> ("Array OUT"=w303:dbl[])  [unwired: 3 in, 1 out]
                      n184 = Absolute Value(x=w303) -> (abs(x)=w302:dbl[])
                      n185 = Bundle(w302, w315) -> (w311:cluster{dbl[], dbl[]})  [unwired: 1 in]
                      n186 = property on="Igraph" class="XYGraph (strict)"() -> ("YScale.Mapping Mode"=w306:u8)  [unwired: 2 in, 2 out]
                      n187 = local write "Igraph"(w311) -> ()
                      n188 = property on="Igraph" class="XYGraph (strict)"("YScale.Minimum"=w306) -> ()  [unwired: 2 in, 2 out]
                    }
                  }
                  n189 = Subtract(x=w301, y=w296) -> (x-y=w278:dbl)
                  n190 = Subtract(x=w295, y=w278) -> (x-y=w277:dbl)
                  n191 = Greater Than 0?(x=w277) -> (x > 0?=w279:bool)
                  n192 = Format Into String(format string="%d", w277) -> (resulting string=w299:string)  [unwired: 2 in, 1 out]
                  n193 = local read "abort"() -> (w294:bool)
                  n194 = Not(x=w294) -> (.not. x?=w300:bool)
                  n195 = And(x=w279, y=w300) -> (x .and. y?=w297:bool)
                  n196 = Concatenate Strings(w283, "\r\n", "Timer status: ", w299) -> (w293:string)
                  n197 = local write "STATUS 1"(w293) -> ()
                  n198 = Wait (ms)(milliseconds to wait=u32 100) -> ()  [unwired: 1 out]
                }
              }
              frame #1 {
                # "Read and Update IV plot and T/RH with the new measurement and increment voltage for the new measurement step"
                n199 = local read "abort"() -> (w335:bool)
                n200 = case shown="False" w335 {
                  tunnel: [w348 w501] -> w336
                  tunnel: w337 -> [w347 _]
                  tunnel: w338 -> [w346 _]
                  tunnel: [w344 w501] -> w339
                  tunnel: w340 -> [w345 _]
                  tunnel: [w343 w501] -> w334
                  tunnel: w333 -> [w342 w500]
                  tunnel: [w341 w500] -> w332
                  frame False {
                    # "\"ABORT\" button NOT pressed"
                    n201 = stacked-sequence {
                      seq-local: [w350 _ _] -> [_ w405 _]
                      seq-local: [w368 _ _] -> [_ _ w466]
                      seq-local: [w367 _ _] -> [_ _ w467]
                      tunnel: w345 -> [_ w402 w472]
                      tunnel: w346 -> [_ _ w464]
                      tunnel: [_ _ w470] -> w348
                      tunnel: [_ _ w469] -> w344
                      tunnel: w347 -> [_ _ _]
                      tunnel: [w374 _ _] -> w343
                      tunnel: w342 -> [_ w403 w458]
                      tunnel: [_ _ w457] -> w341
                      frame #0 {
                        # "Write Relative Humidity [%] in 4th column"
                        # "Write Temperature [ºC] in 3rd column"
                        # "Write Current [nA] in 2nd column"
                        # "Write Voltage [V] in 1st column"
                        # "Increase in 1 the measurement number"
                        # "Convert to nA"
                        # "Show \"Reading current ...\" message \nin \"Current status:\" indicator"
                        # "Show date/time of last measurement \nin \"Last reading at:\" indicator"
                        # "READ and WRITE Voltage/Current/Temperature/Relative Humidity. Check compliance. Show date/time of last measurement and \"Reading current...\" message."
                        n202 = global read "QC_MeasurementSetup.vi" "IV Measurement Parameters"() -> (w366:T10)
                        n203 = Get Date/Time String(want seconds? (F)=TRUE) -> (time string=w371:string)  [unwired: 2 in, 1 out]
                        n204 = local write "Last reading at:"(w371) -> ()
                        n205 = local write "STATUS 1"("Reading current ..." ("status")) -> ()
                        n206 = Unbundle By Name(w366) -> ("Supply"=w361:refnum<class "SupplyControl.lvclass">, "Set Current Limit?"=w365:bool, "Current Limit [µA]"=w363:dbl, "Arduino"=w359:refnum<class "ArduinoControl.lvclass">, "Temperature Readout"=w360:enum16{"Read Arduino", "Enter manually"})
                        n207 = call-dynamic "Supply_ReadCurrent.vi"("SupplyControl in"=w361) -> ("error out"=w367:errorcluster, "Current in nA"=w375:dbl, "SupplyControl out"=w368:refnum<class "SupplyControl.lvclass">)  [unwired: 8 in]
                        n208 = Multiply(x=w363, y=1000.0) -> (x*y=w362:dbl)
                        n209 = case shown="True" w365 {
                          tunnel: w375 -> [_ w395]
                          tunnel: w362 -> [_ w393]
                          tunnel: [FALSE w392] -> w374
                          frame False {
                            # "Measurement without compliance"
                          }
                          frame True {
                            # "Current > Compliance?"
                            n210 = Absolute Value(x=w395) -> (abs(x)=w394:dbl)
                            n211 = Greater?(x=w394, y=w393) -> (0:w392:bool)
                          }
                        }
                        n212 = case shown="\"Read Arduino\"" w360 {
                          tunnel: [w384 w390] -> w372
                          tunnel: [w381 w389] -> w369
                          tunnel: w359 -> [_ w388]
                          frame "Enter manually", Default {
                            # "Read T/RH entered manually"
                            n213 = local read "Temp."() -> (w386:dbl[])
                            n214 = local read "RH"() -> (w382:dbl[])
                            n215 = Index Array(array=w386, index=0) -> (element=w384:dbl)
                            n216 = Index Array(array=w382, index=0) -> (element=w381:dbl)
                          }
                          frame "Read Arduino" {
                            # "Read  T/RH from Arduino"
                            n217 = call "ArduinoRead.vi"("Arduino function"=enum16{"T/RH", "Interlock", "Edgesense"}."T/RH", "ArduinoControl in"=w388) -> ("rel. Humidity [%]"=w389:dbl, "Temperature [°C]"=w390:dbl)  [unwired: 4 in, 4 out]
                          }
                        }
                        n218 = local read "Current reading No."() -> (w355:u32)
                        n219 = local read "Current reading No."() -> (w349:u32)
                        n220 = local read "Current reading No."() -> (w357:u32)
                        n221 = local read "Current reading No."() -> (w356:u32)
                        n222 = local read "Current Volts:"() -> (w376:dbl)
                        n223 = local read "Current reading No."() -> (w351:u32)
                        n224 = call "IVData.vi"("Action"=T3."Write Element", "Array No."=u32 2, "Array Size / Index"=w355, "Data IN"=w372) -> ()  [unwired: 1 in, 2 out]
                        n225 = call "IVData.vi"("Action"=T3."Write Element", "Array No."=u32 3, "Array Size / Index"=w349, "Data IN"=w369) -> ()  [unwired: 1 in, 2 out]
                        n226 = call "IVData.vi"("Action"=T3."Write Element", "Array No."=0, "Array Size / Index"=w357, "Data IN"=w376) -> ()  [unwired: 1 in, 2 out]
                        n227 = call "IVData.vi"("Action"=T3."Write Element", "Array No."=u32 1, "Array Size / Index"=w356, "Data IN"=w375) -> ()  [unwired: 1 in, 2 out]
                        n228 = Increment(x=w351) -> (x+1=w350:u32)
                        n229 = local write "Current reading No."(w350) -> ()
                      }
                      frame #1 {
                        w398 = T3."Read Array" ("Action")
                        w415 = u32 5 ("y")
                        # "Update Current/Voltage plots"
                        # "Set minimum in Current (Y) axis in 0 if linear and 1 if logarithmic"
                        # "Update IV plot and show Temperature/Relative Humidity and last 5 readings of Current/Voltage"
                        n230 = Greater Than 0?(x=w403) -> (x > 0?=w404:bool)
                        n231 = Select(t=0.01, s=w404, f=w402) -> (s? t:f=w401:dbl)
                        n232 = call "IVData.vi"("Action"=w398, "Array No."=0) -> ("Array OUT"=w397:dbl[])  [unwired: 3 in, 1 out]
                        n233 = call "IVData.vi"("Action"=w398, "Array No."=1) -> ("Array OUT"=w417:dbl[])  [unwired: 3 in, 1 out]
                        n234 = Absolute Value(x=w401) -> ()  [unwired: 1 out]
                        n235 = Absolute Value(x=w397) -> (abs(x)=w396:dbl[])
                        n236 = Array Subset(array=w417, index=0, length=w405) -> (w410:dbl[])
                        n237 = Greater?(x=w405, y=w415) -> (0:w414:bool)
                        n238 = local read "Iscale"() -> (w416:enum16{"nanoAmps", "microAmps", "milliAmps"})
                        n239 = Absolute Value(x=w410) -> (abs(x)=w409:dbl[])
                        n240 = case shown="False" w414 {
                          tunnel: w405 -> [w421 w424]
                          tunnel: w415 -> [_ w423]
                          tunnel: [w421 w423] -> w413
                          tunnel: [0 w422] -> w411
                          frame False {
                          }
                          frame True {
                            n241 = Subtract(x=w424, y=w423) -> (x-y=w422:u32)
                          }
                        }
                        n242 = property on="Igraph" class="XYGraph (strict)"() -> ("YScale.Mapping Mode"=w406:u8)  [unwired: 2 in, 2 out]
                        n243 = case shown="..\"nanoAmps\"" w416 {
                          tunnel: [w449 w450 w453] -> w419
                          tunnel: w409 -> [w449 w452 w455]
                          frame .."nanoAmps" {
                          }
                          frame "microAmps" {
                            # "Converts nA to µA"
                            n244 = Divide(x=w452, y=1000.0) -> (x/y=w450:dbl[])
                          }
                          frame "milliAmps".. {
                            # "Converts nA to mA"
                            n245 = Divide(x=w455, y=1000000.0) -> (x/y=w453:dbl[])
                          }
                        }
                        n246 = property on="Igraph" class="XYGraph (strict)"("YScale.Minimum"=w406) -> ()  [unwired: 2 in, 2 out]
                        n247 = for {
                          N: 4 -> [_]
                          tunnel: w413 -> [w429]
                          tunnel: w411 -> [w428]
                          tunnel: w405 -> [w425]
                          i -> [w430]
                          # "Update \"Last 5 readings:\" IV indicator and T/RH indicators"
                          n248 = call "IVData.vi"("Action"=T3."Read Array", "Array No."=w430) -> ("Array OUT"=w427:dbl[])  [unwired: 3 in, 1 out]
                          n249 = case shown="3.." w430 {
                            tunnel: w429 -> [w433 w437 _ _]
                            tunnel: w428 -> [w434 w438 _ _]
                            tunnel: w427 -> [w432 w436 w442 w447]
                            tunnel: w425 -> [_ _ w440 w445]
                            frame ..0 {
                              # "Read Voltage from 1st column"
                              n250 = Array Subset(array=w432, index=w434, length=w433) -> (w431:dbl[])
                              n251 = local write "Volts"(w431) -> ()
                            }
                            frame 1 {
                              # "Read Current from 2nd column"
                              n252 = Array Subset(array=w436, index=w438, length=w437) -> (w435:dbl[])
                              n253 = local write "Current"(w435) -> ()
                            }
                            frame 2 {
                              # "Read Temperature from 3rd column"
                              n254 = Decrement(x=w440) -> (x-1=w439:u32)
                              n255 = Array Subset(array=w442, index=w439, length=1) -> (w441:dbl[])
                              n256 = local write "Temp."(w441) -> ()
                            }
                            frame 3.. {
                              # "Read Relative Humidity from 4th column"
                              n257 = Decrement(x=w445) -> (x-1=w444:u32)
                              n258 = Array Subset(array=w447, index=w444, length=1) -> (w446:dbl[])
                              n259 = local write "RH"(w446) -> ()
                            }
                          }
                        }
                        n260 = Bundle(w396, w419) -> (w407:cluster{dbl[], dbl[]})  [unwired: 1 in]
                        n261 = local write "Igraph"(w407) -> ()
                      }
                      frame #2 {
                        # "Increase volts and check for end of ramp"
                        # "Increase voltage and check compliance"
                        n262 = local read "Current Volts:"() -> (w459:dbl)
                        n263 = local read "Current Volts:"() -> (w456:dbl)
                        n264 = local read "positive ramp?"() -> (w468:bool)
                        n265 = Quotient & Remainder(x=w456, y=w464) -> (x-y*floor(x/y)=w465:dbl, floor(x/y)=w463:dbl)
                        n266 = case shown="False" w468 {
                          tunnel: w464 -> [w475 w479]
                          tunnel: w472 -> [w476 w482]
                          tunnel: [w474 w481] -> w460
                          tunnel: [w473 w478] -> w471
                          tunnel: w459 -> [w477 w480]
                          frame False {
                            n267 = Subtract(x=w477, y=w476) -> (x-y=w473:dbl)
                            n268 = Greater Or Equal?(x=w473, y=w475) -> (x >= y?=w474:bool)
                          }
                          frame True {
                            n269 = Add(x=w480, y=w482) -> (x+y=w478:dbl)
                            n270 = Less Or Equal?(x=w478, y=w479) -> (x <= y?=w481:bool)
                          }
                        }
                        n271 = Not Equal To 0?(x=w465) -> (x != 0?=w461:bool)
                        n272 = Equal To 0?(x=w463) -> (x = 0?=w462:bool)
                        n273 = Or(x=w461, y=w462) -> ()  [unwired: 1 out]
                        n274 = case shown="False" w460 {
                          tunnel: w471 -> [_ w497]
                          tunnel: [w485 FALSE] -> w470
                          tunnel: [FALSE w487] -> w469
                          tunnel: w456 -> [_ w495]
                          tunnel: w467 -> [_ w494]
                          tunnel: w466 -> [_ w493]
                          tunnel: w458 -> [w484 _]
                          tunnel: [w483 0] -> w457
                          frame False {
                            (unwired) TRUE
                            n275 = Increment(x=w484) -> (x+1=w483:i32)
                            n276 = Greater Or Equal?(x=w484) -> (x >= y?=w485:bool)  [unwired: 1 in]
                          }
                          frame True {
                            # "Message \"Incrementing volts.\""
                            # "Increase  voltage, check compliance and check PTP supply errors"
                            n277 = local read "step [V]"() -> (w491:dbl)
                            n278 = call "SupplyRamp.vi"("error in"=w494, "Requested Voltage"=w497, "Step Size"=w491, "Step Delay"=100, "Supply IN"=w493, "Starting Voltage"=w495) -> ("error out"=w489:errorcluster, "Compliance exceeded"=w487:bool, "Current Voltage"=w492:dbl)  [unwired: 2 in, 1 out]
                            n279 = local write "STATUS 1"("Incrementing volts.") -> ()
                            n280 = case shown="No Error" w489 {
                              tunnel: w492 -> [w499 _]
                              frame No Error {
                                n281 = local write "Current Volts:"(w499) -> ()
                              }
                              frame Error {
                              }
                            }
                            n282 = property on="Bias On/Off:" class="Bool (strict)"("Blinking"=w487) -> ()  [unwired: 2 in, 2 out]
                          }
                        }
                      }
                    }
                  }
                  frame True {
                    w501 = FALSE
                    # "\"ABORT\" button pressed"
                  }
                }
              }
            }
            n283 = case shown="False" w252 {
              frame False {
              }
              frame True {
                n284 = property on="Bias On/Off:" class="Bool (strict)"("Blinking"=TRUE) -> ()  [unwired: 2 in, 2 out]
              }
            }
            n285 = Build Array(w253, w252, "abort", w248) -> (w257:bool[])
            n286 = Or Array Elements(Boolean array=w257) -> (logical OR=w263:bool)
            n287 = Not(x=w263) -> (.not. x?=w262:bool)
          }
        }
        frame True {
          w503 = FALSE
          # "Flag compliance as reason for end of run"
          # "Compliance exceeded when first voltage applied"
          n288 = local write "STATUS 1"("Run aborted - compliance exceeded.") -> ()
          n289 = Build Array(w503, TRUE, w503, w503) -> (w504:bool[])
        }
      }
      n290 = Search 1D Array(1D array=w237, element=TRUE) -> (index of element=w235:i32)  [unwired: 1 in]
      n291 = Increment(x=w235) -> (x+1=w234:i32)
      n292 = case shown="1" w234 {
        tunnel: ["" "Run ended normally" "Compliance exceeded" "Run aborted - by user" "Run aborted - Ilimit exceeded"] -> w229
        frame ..0 {
        }
        frame 1 {
        }
        frame 2 {
        }
        frame 3 {
        }
        frame 4.. {
        }
      }
      n293 = Concatenate Strings(w229, "\r\n", "RAMPING DOWN VOLTS") -> (w232:string)
      n294 = global read "QC_RunInformation.vi" "Run info"() -> (w233:T7)
      n295 = Bundle By Name(cluster=w233, "End of Run comment:"=w229) -> (w228:T7)
      n296 = local write "STATUS 1"(w232) -> ()
      n297 = global write "QC_RunInformation.vi" "Run info"(w228) -> ()
    }
    frame #4 {
      # "Ramp down, switch off supply, ask to save data and save jpg of the Front Panel"
      n298 = stacked-sequence {
        frame #0 {
          # "Switch IV supply to STANDBY"
          # "s -> ms"
          # "Ramp down voltage and switch IV supply to standby"
          n299 = global read "QC_MeasurementSetup.vi" "IV Measurement Parameters"() -> (w515:T10)
          n300 = Unbundle By Name(w515) -> ("Supply"=w514:refnum<class "SupplyControl.lvclass">, "Ramp down Interval [s]"=w507:i32, "Ramp down steps [V]"=w508:dbl, "Switching"=w509:refnum<class "Switching.lvclass">, "Matrix used?"=w510:bool)
          n301 = local read "Current Volts:"() -> (w520:dbl)
          n302 = Multiply(x=w507, y=1000) -> (x*y=w517:i32)
          n303 = call "SupplyRamp.vi"("Requested Voltage"=0.0, "Step Size"=w508, "Step Delay"=w517, "Supply IN"=w514, "Starting Voltage"=w520) -> ("error out"=w513:errorcluster, "Supply OUT"=w512:refnum<class "SupplyControl.lvclass">, "Current Voltage"=w518:dbl)  [unwired: 3 in, 1 out]
          n304 = local write "Current Volts:"(w518) -> ()
          n305 = call-dynamic "Supply_Stby.vi"("error in (no error)"=w513, "SupplyControl in"=w512) -> ("error out"=w511:errorcluster)  [unwired: 8 in, 1 out]
          n306 = case shown="True" w510 {
            tunnel: w509 -> [_ w525]
            tunnel: w511 -> [_ w524]
            frame False {
            }
            frame True {
              # "CLOSE Switching Matrix"
              # "RESET Switching  Matrix"
              n307 = call-dynamic "MatrixSwitch.vi"("error in (no error)"=w524, "Action"=T4."Reset", "Switching in"=w525) -> ("error out"=w521:errorcluster, "Switching out"=w522:refnum<class "Switching.lvclass">)  [unwired: 6 in, 1 out]
              n308 = call-dynamic "Close.vi"("error in (no error)"=w521, "Switching in"=w522) -> ()  [unwired: 8 in, 2 out]
            }
          }
        }
        frame #1 {
          w530 = 0
          # "\"Current Volts\" indicator back to 0.00 V"
          # "\"Bias  On/Off\" indicator in Off (red)"
          # "\"ABORT\" button disanabled \nand dimmed (Disabled=2)"
          # "\"QUIT\" and \"Save & QUIT\" buttons \nenabled (Disabled=0)"
          # "Reset \"Current Volts\" and \"Bias On/Off\" indicators, \"ABORT\" button disabled and \"QUIT\"/\"Save & QUIT\" buttons enabled"
          n309 = property on="Quit & Save" class="Bool"("DisabledEnum"=w530) -> ()  [unwired: 2 in, 2 out]
          n310 = property on="quit (no save)" class="Bool"("DisabledEnum"=w530) -> ()  [unwired: 2 in, 2 out]
          n311 = local write "Current Volts:"(0.0 ("Current Volts:")) -> ()
          n312 = property on="abort" class="Bool (strict)"("DisabledEnum"=2) -> ()  [unwired: 2 in, 2 out]
          n313 = local write "Bias On/Off:"(FALSE ("Visible")) -> ()
          n314 = local write "STATUS 1"("Run finished. \nSave data?" ("STATUS 1")) -> ()
        }
        frame #2 {
          # "Save  jpg  image of the Front Panel"
          n315 = Current VI's Path() -> (path=w532:path)
          n316 = call "SaveJPEG.vi"("Test"="IV", "File Path Control"=w532) -> ()  [unwired: 1 in, 2 out]
        }
      }
    }
    frame #5 {
      # "*WARNING*: \"Done!\" indicator in \nFront Panel hidden."
      # "Switch off Arduino if used for T/RH measurement"
      # "Display and save data"
      n317 = local read "Scales"() -> (w543:T1)
      n318 = global read "QC_MeasurementSetup.vi" "IV Measurement Parameters"() -> (w541:T10)
      n319 = local read "Iscale"() -> (w542:enum16{"nanoAmps", "microAmps", "milliAmps"})
      n320 = while {
        shift-left: w542 -> [w588]
        shift-right: [w587] -> _
        shift-left: w543 -> [w590]
        shift-right: [w589] -> _
        tunnel: ["Quit & Save"] -> w545
        tunnel: ["quit (no save)"] -> w544
        stop <- w585 continue-if-true
        # "Loop and await decision on whether to save or junk data"
        n321 = local read "Scales"() -> (w589:T1)
        n322 = local read "Iscale"() -> (w587:enum16{"nanoAmps", "microAmps", "milliAmps"})
        n323 = Not Equal?(x=w590, y=w589) -> (x != y?=w583:bool)
        n324 = Not Equal?(x=w588, y=w587) -> (x != y?=w582:bool)
        n325 = case shown="True" w583 {
          tunnel: w589 -> [_ w617]
          frame False {
          }
          frame True {
            # "Allow to change the IV plot representation (Linear=0, Logarithmic=1)"
            n326 = case shown="..\"Lin - Lin\"" w617 {
              tunnel: [w618 1 0 w623] -> w616
              tunnel: [w618 0 1 w623] -> w615
              frame .."Lin - Lin" {
                w618 = 0
              }
              frame "Log - Lin" {
              }
              frame "Lin - Log" {
              }
              frame "Log - log".. {
                w623 = 1
              }
            }
            n327 = property on="Igraph" class="XYGraph (strict)"("X Scale.Mapping Mode"=w616) -> ()  [unwired: 2 in, 2 out]
            n328 = property on="Igraph" class="XYGraph (strict)"("Y Scale.Mapping Mode"=w615, "YScale.Minimum"=w615) -> ()  [unwired: 2 in, 2 out]
          }
        }
        n329 = case shown="True" w582 {
          tunnel: w587 -> [_ w603]
          frame False {
          }
          frame True {
            w596 = T3."Read Array" ("Action")
            # "Set minimum in Current (Y) axis in 0 if linear and 1 if logarithmic"
            # "Allow to change the Current scale (nA, µA or mA)"
            n330 = global read "QC_MeasurementSetup.vi" "IV Measurement Parameters"() -> (w598:T10)
            n331 = property on="Igraph" class="XYGraph (strict)"() -> ("YScale.Mapping Mode"=w599:u8)  [unwired: 2 in, 2 out]
            n332 = property on="Igraph" class="XYGraph (strict)"("YScale.Minimum"=w599) -> ()  [unwired: 2 in, 2 out]
            n333 = Unbundle By Name(w598) -> ("Number Of Steps"=w595:u32)
            n334 = local read item#-1() -> (w594)
            n335 = Add(x=w595, y=w594) -> (x+y=w593:u32)
            n336 = call "IVData.vi"("Action"=w596, "Array No."=u32 1 ("Action")) -> ("Array OUT"=w605:dbl[])  [unwired: 3 in, 1 out]
            n337 = Array Subset(array=w605, index=0, length=w593) -> (w602:dbl[])
            n338 = Absolute Value(x=w602) -> (abs(x)=w601:dbl[])
            n339 = call "IVData.vi"("Action"=w596, "Array No."=u32 0 ("Action")) -> ("Array OUT"=w592:dbl[])  [unwired: 3 in, 1 out]
            n340 = case shown="\"microAmps\"" w603 {
              tunnel: [w608 w609 w613] -> w607
              tunnel: w601 -> [w608 w611 w614]
              frame .."nanoAmps" {
              }
              frame "microAmps" {
                n341 = Divide(x=w611, y=1000.0) -> (x/y=w609:dbl[])
              }
              frame "milliAmps".. {
                n342 = Divide(x=w614, y=1000000.0) -> (x/y=w613:dbl[])
              }
            }
            n343 = Absolute Value(x=w592) -> (abs(x)=w591:dbl[])
            n344 = Bundle(w591, w607) -> (w604:cluster{dbl[], dbl[]})  [unwired: 1 in]
            n345 = local write "Igraph"(w604) -> ()
          }
        }
        n346 = Not Or(1:"quit (no save)", 2:"Quit & Save") -> (0:w585:bool)
      }
      n347 = Unbundle By Name(w541) -> ("Temperature Readout"=w540:enum16{"Read Arduino", "Enter manually"}, "Arduino"=w534:refnum<class "ArduinoControl.lvclass">)
      n348 = case shown="\"Read Arduino\"" w540 {
        tunnel: w534 -> [_ w581]
        frame "Enter manually", Default {
        }
        frame "Read Arduino" {
          n349 = call "ArduinoClose.vi"("ArduinoControl in"=w581) -> ()  [unwired: 9 in, 2 out]
        }
      }
      n350 = case shown="True" w544 {
        tunnel: [FALSE w625] -> w546
        frame False {
        }
        frame True {
          n351 = Two Button Dialog(message="Are you sure you don't want to save the data?", 1:"Quit" ("F button name (\"Cancel\")"), 2:"Save data" ("T button name (\"OK\")")) -> (T button?=w625:bool)
        }
      }
      n352 = Or(x=w545, y=w546) -> (x .or. y?=w539:bool)
      n353 = flat-sequence {
        tunnel: w539 -> [w549]
        tunnel: [w549] -> w535
        tunnel: [TRUE] -> w533
        frame #0 {
          # "Extract breakdown voltage"
          n354 = global read "QC_MeasurementSetup.vi" "IV Measurement Parameters"() -> (w558:T10)
          n355 = Unbundle By Name(w558) -> ("V_breakdown Limit [V]"=w552:dbl, "Number Of Steps"=w553:u32)
          n356 = call "ScanFeedback.vi"("measurement type"=T5."IV") -> ("V breakdown"=w547:dbl)  [unwired: 4 in, 4 out]
          n357 = Absolute Value(x=w547) -> (abs(x)=w550:dbl)
          n358 = Absolute Value(x=w552) -> (abs(x)=w551:dbl)
          n359 = Greater Or Equal?(x=w550, y=w551) -> (x >= y?=w554:bool)
          n360 = case shown="True" w549 {
            tunnel: ["" w580] -> w559
            tunnel: [_ w565] -> w557
            tunnel: w553 -> [_ w563]
            frame False {
            }
            frame True {
              w576 = T3."Read Array" ("Action")
              # "Show \"Saving Data ...\" message"
              # "Save data in file"
              n361 = local read item#-1() -> (w562)
              n362 = local write "STATUS 1"("Saving Data ...") -> ()
              n363 = Add(x=w563, y=w562) -> ()  [unwired: 1 out]
              n364 = call "IVData.vi"("Action"=w576, "Array No."=u32 0 ("Action")) -> ("Array OUT"=w571:dbl[])  [unwired: 3 in, 1 out]
              n365 = call "IVData.vi"("Action"=w576, "Array No."=u32 1 ("Action")) -> ("Array OUT"=w570:dbl[])  [unwired: 3 in, 1 out]
              n366 = Build Array(w571, w570) -> (w569:dbl[][])
              n367 = Transpose 2D Array(2D array=w569) -> (transposed array=w568:dbl[][])
              n368 = call "IVData.vi"("Action"=w576, "Array No."=u32 3 ("Action")) -> ("Array OUT"=w578:dbl[])  [unwired: 3 in, 1 out]
              n369 = call "IVData.vi"("Action"=w576, "Array No."=u32 2 ("Action")) -> ("Array OUT"=w577:dbl[])  [unwired: 3 in, 1 out]
              n370 = call <vilib>:"Std Deviation and Variance.vi"("X"=w578) -> ("mean"=w566:dbl)  [unwired: 1 in, 2 out]
              n371 = call <vilib>:"Std Deviation and Variance.vi"("X"=w577) -> ("mean"=w567:dbl)  [unwired: 1 in, 2 out]
              n372 = call "SaveDataFile.vi"("Data Array"=w568, "Temperature"=w567, "Humidity"=w566, "Array Titles"="Voltage[V] Current[nA]\n", "Strip Segment"="") -> ("Path + Filename OUT"=w580:string, "Error Out"=w565:errorcluster)  [unwired: 7 in, 2 out]
            }
          }
          n373 = call "WriteLogFile.vi"("Automatic warning"="", "Data File"=w559, "Error In"=w557, "DUT passed?"=w554, "Value TechSpec criteria"=w547, "Files saved?"=w549) -> ()  [unwired: 5 in, 1 out]
        }
      }
      n374 = Select(t="Run finished.\nData saved." ("STATUS 1"), s=w535, f="Run finished.\nData not saved." ("STATUS 1")) -> (s? t:f=w538:string)
      n375 = local write "STATUS 1"(w538) -> ()
      "Done!" <- w533
    }
  }
